vi "GetVelocity.vi"(8 "error in (no error)":errorcluster, 11 "VISA resource name":refnum<visa-resource-name>) -> (0 "error out":errorcluster, 2 "Velocity":dbl)   [LabVIEW 2014, in "GRBLMotionCore.lvlib"]
doc: "Performs an instrument error query before terminating the software connection to the instrument."
uses:
  <instrlib>/GRBL/GRBLMotionCore.lvlib
  <vilib>/Utility/error.llb/DialogType.ctl
  <vilib>/regexp/Match Regular Expression.xnode
panel:
  out "Read Buffer":string
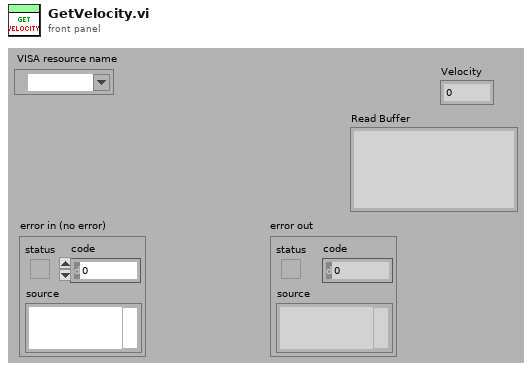
[diagram p1: front panel]
types:
  T1 = typedef "DialogType.ctl" = u16
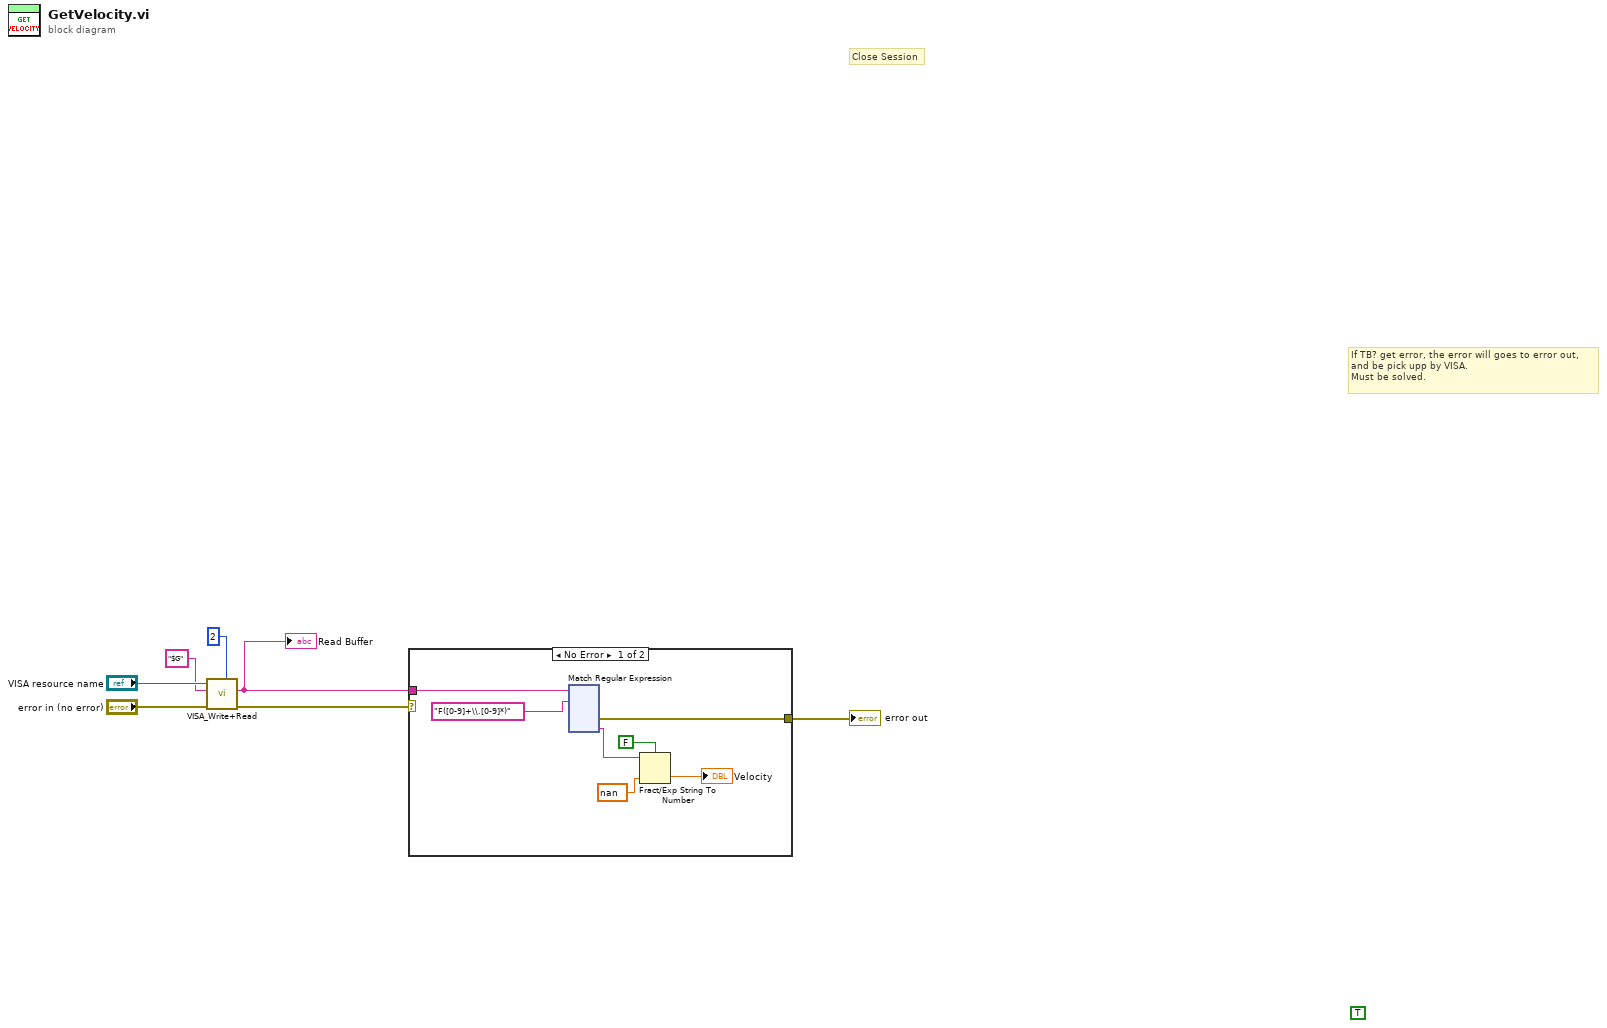
[diagram p0: block diagram]
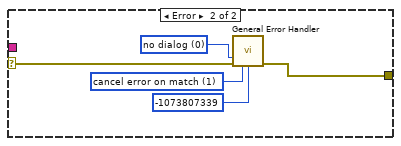
[diagram p2: hidden frame]
diagram:
  (unwired) TRUE
  # "If TB? get error, the error will goes to error out, \nand be pick upp by VISA.\nMust be solved."
  # "Close Session"
  n1 = call <instrlib>:"VISA_Write+Read.vi"("NumRead"=2, "error in (no error)"="error in (no error)", "Write Buffer"="$G" ("string"), "VISA resource name"="VISA resource name") -> ("error out"=w3:errorcluster, "readout"=w4:string)  [unwired: 5 in, 1 out]
  "Read Buffer" <- w4
  n2 = case shown="No Error" w3 {
    selector: w3 -> [_ w130]
    tunnel: w4 -> [w11 _]
    tunnel: [w8 w129] -> w2
    frame No Error {
      n3 = xnode "Match Regular Expression"("input string"=w11, "regular expression"="F([0-9]+\\.[0-9]*)") -> ("error out"=w8:errorcluster, "submatch 1"=w13:string)  [unwired: 4 in, 4 out]
      n4 = Fract/Exp String To Number(use system decimal point (T)=FALSE, string=w13, default (0 dbl)=nan ("default value 1")) -> (number=→"Velocity":dbl)  [unwired: 1 in, 1 out]
    }
    frame Error {
      w128 = T1 0 items=["no dialog", "OK message", "continue or stop message", "OK message + warnings", "continue/stop + warnings"] ("type of dialog (OK msg:1)")
      w132 = 1 items=["no exception", "cancel error on match", "set error on match"] ("[exception action] (none:0)")
      n5 = call <vilib>:"General Error Handler.vi"("type of dialog (OK msg:1)"=w128, "error in (no error)"=w130, "[exception action] (none:0)"=w132, "[exception code]"=-1073807339) -> ("error out"=w129:errorcluster)  [unwired: 7 in, 4 out]
    }
  }
  "error out" <- w2
